vi "VALVE_return_valve_position.vi"(4 "error in":errorcluster, 7 "Valves positions":u8[](array[numeric])) -> (0 "error out":errorcluster, 3 "Position":u8)   [LabVIEW 2015]
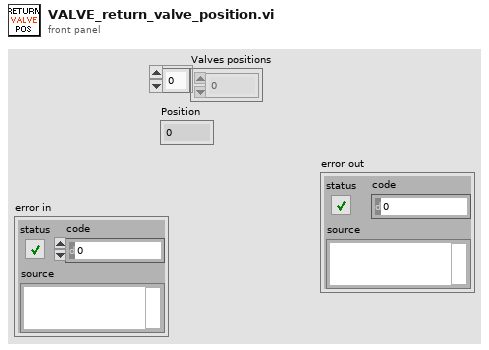
[diagram p1: front panel]
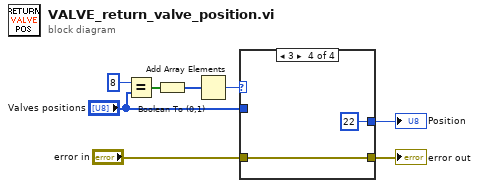
[diagram p0: block diagram]
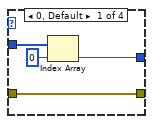
[diagram p2: hidden frame]
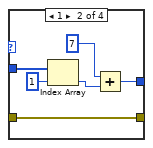
[diagram p3: hidden frame]
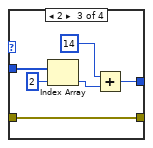
[diagram p4: hidden frame]
diagram:
  n1 = Equal?(x=u8 8 ("Position"), y="Valves positions") -> (x = y?=w7:bool[])
  n2 = Boolean To (0,1)(Boolean=w7) -> (0, 1=w6:i16[])
  n3 = Add Array Elements(numeric array=w6) -> (sum=w5:i16)
  n4 = case shown="3" w5 {
    tunnel: "Valves positions" -> [w12 w18 w24 _]
    tunnel: [w10 w15 w21 u8 22 ("Valve position OUT")] -> w3
    tunnel: "error in" -> [w9 w13 w19 w26]
    tunnel: [w9 w13 w19 w26] -> w1
    frame 0, Default {
      n5 = Index Array(array=w12, index=0) -> (element=w10:u8)
    }
    frame 1 {
      n6 = Index Array(array=w18, index=1) -> (element=w16:u8)
      n7 = Add(x=u8 7, y=w16) -> (x+y=w15:u8)
    }
    frame 2 {
      n8 = Index Array(array=w24, index=2) -> (element=w22:u8)
      n9 = Add(x=u8 14, y=w22) -> (x+y=w21:u8)
    }
    frame 3 {
    }
  }
  "Position" <- w3
  "error out" <- w1
